vi "Test Prepare.vi"(0 "reference in":refnum<class "Test.lvclass">, 5 "error in (no error)":errorcluster) -> (14 "reference out":refnum<class "Test.lvclass">, 19 "error out":errorcluster)   [LabVIEW 2013, in "Test.lvclass"]
uses:
  Test.lvclass
  Device_class/Device.lvclass
  Temp_class/Temp.lvclass
  Torque_class/Torque.lvclass
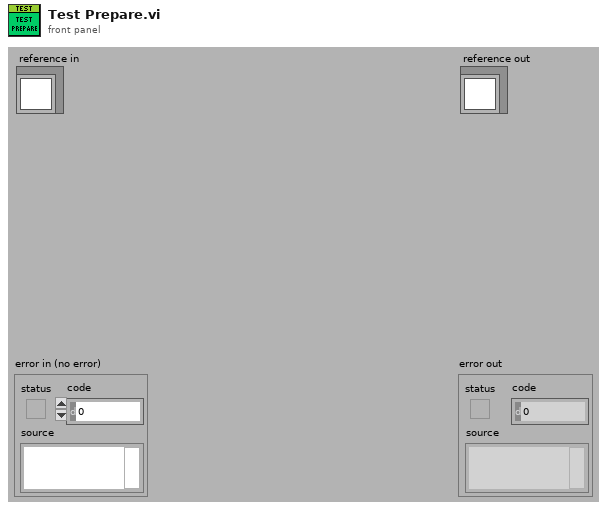
[diagram p1: front panel]
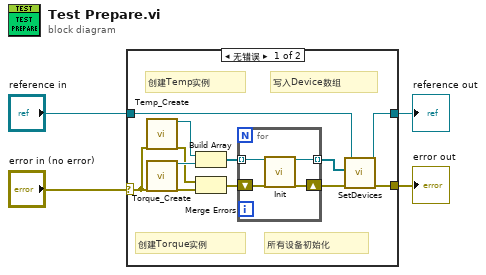
[diagram p0: block diagram]
diagram:
  n1 = case shown="无错误" "error in (no error)" {
    selector: "error in (no error)" -> [w16 w22]
    tunnel: [w6 w22] -> w3
    tunnel: [w5 w21] -> w1
    tunnel: "reference in" -> [w9 w21]
    frame No Error {
      # "写入Device数组"
      # "所有设备初始化"
      # "创建Temp实例"
      # "创建Torque实例"
      n2 = call "Temp_Create.vi"("error in (no error)"=w16) -> ("reference out"=w15:refnum<class "Temp.lvclass">, "error out"=w12:errorcluster)  [unwired: 17 in]
      n3 = call "Torque_Create.vi"("error in (no error)"=w16) -> ("reference out"=w14:refnum<class "Torque.lvclass">, "error out"=w11:errorcluster)  [unwired: 17 in]
      n4 = Build Array(w15, w14) -> (w13:refnum<class "Device.lvclass">[])
      n5 = Merge Errors(w12, w11) -> (w10:errorcluster)
      n6 = for {
        tunnel: w13 -> [w20] mode=indexing
        shift-right: [w18] -> w7
        shift-left: w10 -> [w19]
        tunnel: [w17] -> w8 mode=indexing
        n7 = call-dynamic "Init.vi"("reference in"=w20, "error in (no error)"=w19) -> ("reference out"=w17:refnum<class "Device.lvclass">, "error out"=w18:errorcluster)  [unwired: 16 in]
      }
      n8 = call-dynamic "SetDevices.vi"("error in (no error)"=w7, "Devices"=w8, "reference in"=w9) -> ("error out"=w6:errorcluster, "reference out"=w5:refnum<class "Test.lvclass">)  [unwired: 7 in]
    }
    frame Error {
    }
  }
  "error out" <- w3
  "reference out" <- w1
